vi "convert a bunch of expt folders.vi"(8 "error in (no error)":errorcluster, 11 "Array of expt folders":path[](array[path])) -> (0 "error out":errorcluster, 2 "not itx folder":bool[](array[boolean]), 3 "generated tdms files (w/ metadata)":path[](array[path]))   [LabVIEW 2016]
panel:
  out "current directory":path
  out "iteration":i32
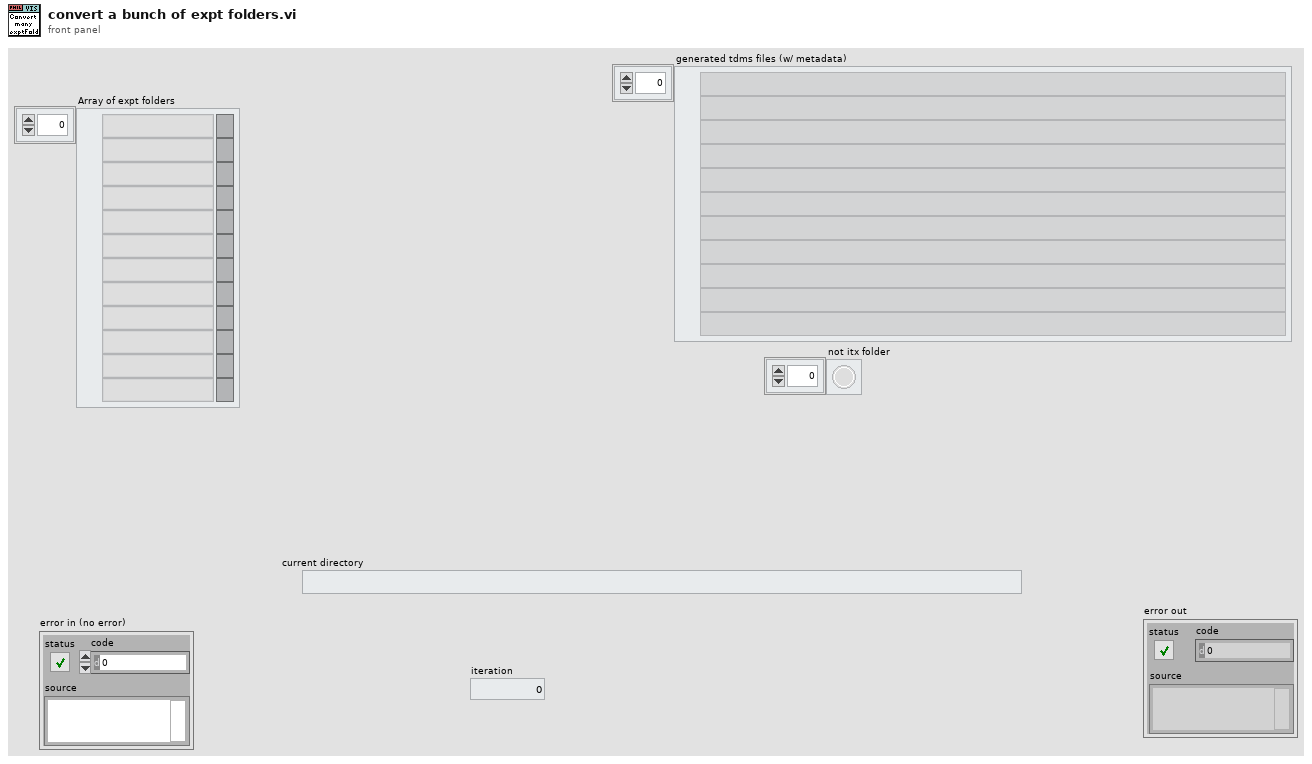
[diagram p1: front panel]
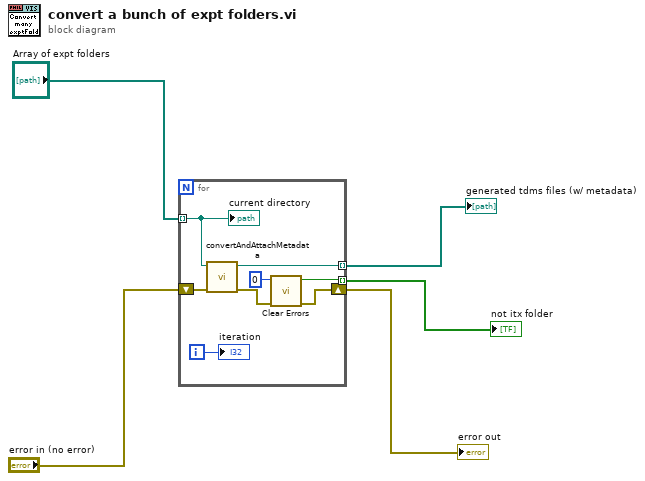
[diagram p0: block diagram]
diagram:
  n1 = for {
    tunnel: "Array of expt folders" -> [w11] mode=indexing
    shift-right: [w8] -> w4
    shift-left: "error in (no error)" -> [w12]
    tunnel: [w10] -> w3 mode=indexing
    tunnel: [w7] -> w1 mode=indexing
    i -> [w13]
    n2 = call "convertAndAttachMetadata.vi"("error in (no error)"=w12, "experiment folder"=w11) -> ("error out"=w9:errorcluster, "generated tdms file path"=w10:path)  [unwired: 8 in]
    n3 = call <vilib>:"Clear Errors.vi"("error in (no error)"=w9, "specific error code to clear (0: all)"=0) -> ("error out"=w8:errorcluster, "specific error cleared?"=w7:bool)  [unwired: 4 in]
    "iteration" <- w13
    "current directory" <- w11
  }
  "error out" <- w4
  "generated tdms files (w/ metadata)" <- w3
  "not itx folder" <- w1
